vi "Detect_Boolean_Change.vi"(0 "NewVal":bool[](array[boolean]), 1 "OldVal":bool[](array[boolean])) -> (2 "FinalVal":bool[](array[boolean]), 3 "SingleEvent":bool, 4 "ButtonId":i32)   [LabVIEW 2012]
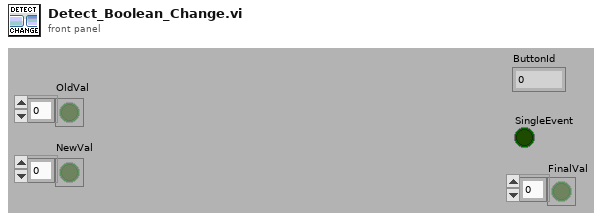
[diagram p1: front panel]
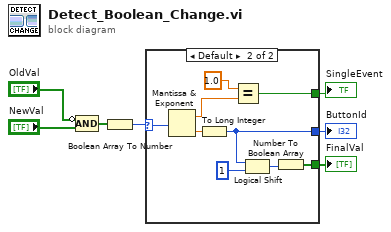
[diagram p0: block diagram]
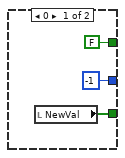
[diagram p2: hidden frame]
diagram:
  n1 = Compound Arithmetic op=AND(invert "OldVal", "NewVal") -> (w5:bool[])
  n2 = Boolean Array To Number(Boolean array=w5) -> (number=w1:u32)
  n3 = case shown="Default" w1 {
    selector: w1 -> [_ w12]
    tunnel: [-1 w18] -> w4
    tunnel: [w8 w15] -> w3
    tunnel: [FALSE w13] -> w2
    frame 0 {
      n4 = local read "NewVal"() -> (w8:bool[])
    }
    frame Default {
      n5 = Mantissa & Exponent(0:w12) -> (1:w14:dbl, 2:w19:dbl)
      n6 = To Long Integer(number=w19) -> (32bit integer=w18:i32)
      n7 = Equal?(x=1.0, y=w14) -> (x = y?=w13:bool)
      n8 = Logical Shift(y=w18, x=1) -> (x << y=w16:i32)
      n9 = Number To Boolean Array(number=w16) -> (Boolean array=w15:bool[])
    }
  }
  "ButtonId" <- w4
  "FinalVal" <- w3
  "SingleEvent" <- w2
